vi "01-QNET_MECHKIT_Flexgage.vi"() -> ()   [LabVIEW 2017]
doc: "This VI is to be used with the NI-ELVIS and the QNET-Mechatronic Sensors I module. The objective is to calibrate the strain gage sensor mounted on the flexible link."
uses:
  <vilib>/Simulation/Scripting/Companion Diagram/SimConfigNode/SimParams.ctl
  <vilib>/Simulation/Scripting/Companion Diagram/SimConfigNode/_simSolvers.ctl
  <vilib>/Simulation/Implementation/Shared/SIMSCR Execution Mode.ctl
  <vilib>/Simulation/Param Hierarchy/Typedefs/SIMPH Param Control Actions.ctl
  <vilib>/Simulation/Implementation/Shared/NILVSim_ParamChanged.vi
  <vilib>/Simulation/Implementation/Shared/NILVSIM_BeginStep.vi
  <vilib>/DAQmx/read.llb/DAQmx Read.vi
  <vilib>/DAQmx/read.llb/DAQmx Read (Analog DBL 1Chan 1Samp).vi
  <vilib>/Simulation/Utility/Implementation/NILVSim Collector.llb/SIM Collector (scalar).vi
  <vilib>/Simulation/SignalDisplay/Implementation/NILVSim Time Waveform.llb/SIM Time Waveform (scalar).vi
  <vilib>/Simulation/Utility/Implementation/SIM Halt.vi
  <vilib>/Simulation/Implementation/Shared/NILVSim_Manager.vi
  <vilib>/Utility/error.llb/Clear Errors.vi
  <vilib>/Simulation/Implementation/Shared/NILVSim_FinalizeModel.vi
  <vilib>/Simulation/Utility/Implementation/NILVSim Collector.llb/NILVSim Collector core (scalar).vi
  <vilib>/Simulation/Implementation/Shared/SIM Unbundle Sim Info.vi
  <vilib>/Simulation/Implementation/Shared/NILVSim_Initialize.vi
  <vilib>/Analysis/6fits.llb/Linear Fit.vi
  <vilib>/DAQmx/miscellaneous.llb/DAQmx Fill In Error Info.vi
  <vilib>/Simulation/Utility/Implementation/NILVSim Get Time and IsAcceptedStep.vi
  <vilib>/Simulation/Implementation/Shared/SIMSH Read Queue.vi
  <vilib>/Simulation/Implementation/Shared/NILVSim_GetModelError.vi
  <vilib>/Simulation/Implementation/Shared/SIM Bundle Sim Info.vi
  <vilib>/express/express analysis/Spectral/Block/exnSpectralBlock spectral measurements power poly.vi
  <vilib>/express/express analysis/Spectral/Block/exnSpectralBlock spectral measurements power WFM.vi
  <vilib>/Simulation/Scripting/Companion Diagram/SimConfigNode/SimDog.xnode
  <vilib>/Simulation/Implementation/XNodeFramework/SimXNode/SimX.xnode
  <vilib>/express/express analysis/Spectral/XNode/ExpressSpectralMeasurementsBlockNode.xnode
  <vilib>/Analysis/NI_AALPro.lvlib
  <vilib>/Simulation/Implementation/Shared/NI_SIM_Implementation.lvlib
panel:
  in  "Sampling Rate (Hz)":dbl=100.0 min=0.0 max=1000.0 step=25.0 format="%.1f"
  in  "Device":tag="Dev1"
  in  "Tab Control":T1(tab)
  out "Flexgage (V)":waveform(dbl)(graph)
  in  "Link Position (cm)":dbl[](array[numeric])=[-1.0, -0.5, 0.0, 0.5, 1.0] format="%.1f"
  in  "Sensor Measurement (V)":dbl[](array[numeric])
  out "slope":dbl format="%_3f"
  out "intercept":dbl format="%_3f"
  out "Sensor Readings":T2(graph)
  in  "Offset (cm)":dbl
  in  "Gain (cm/V)":dbl
  out "Flexgage (cm)":waveform(dbl)(graph)
  out "Flexgage (cm) 2":dbl(slide) scale=-1.0..1.0 scale format="%_2f"
  out "Power Spectrum":cluster{"f0":dbl, "df":dbl, "magnitude":dbl[]}(graph)
  in  "stop":bool
  # "QNET-MECHKIT Strain Gage"
  # "NOTE: Place J7 jumper on \"Strain gage\" setting."
  # "1) Move the flexible link at -1.0 cm\n2) Enter measured flexgage sensor values in \"Sensor Measurement (V)\" array.\n3) Repeat for -0.5 cm, 0 cm, 0.5 cm, and 1.0 cm."
  # "Linear curve fitting results:"
  # "Enter gain and offset value for sensor to measure correct position of the flexible link.\n(e.g. display below should read 0.5 cm when ruler is placed at 0.5 cm)."
  # "y = Gain*x + Offset\nwhere\nx is the sensor voltage \ny is the output in centimeters."
  # "1) Perturb the flexible link manually.\n2) Once it stopped resonating, click on the STOP button to stop running the VI.\n3) The spectrum is shown below."
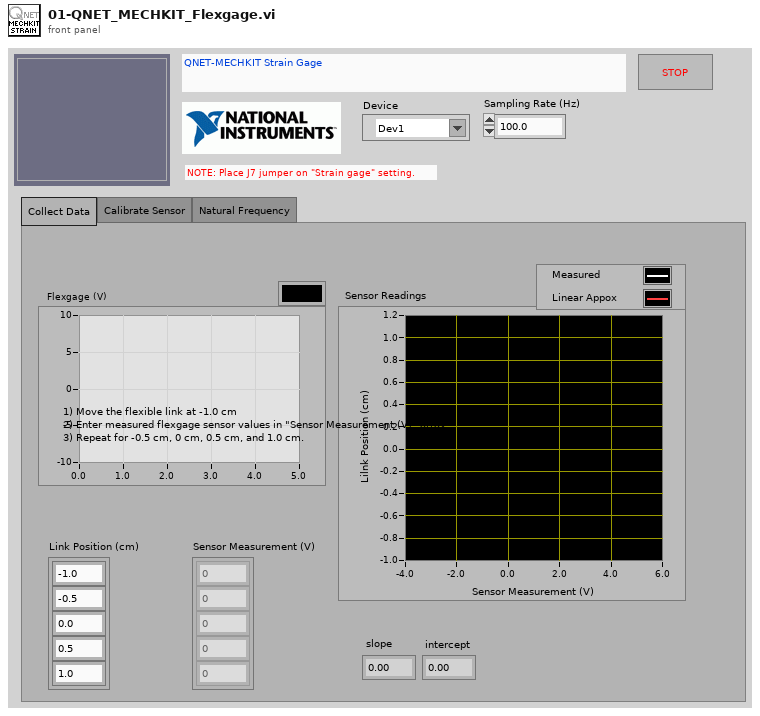
[diagram p1: front panel]
types:
  T1 = enum32{"Collect Data", "Calibrate Sensor", "Natural Frequency"}
  T2 = cluster{"Sensor Measurement (V)":dbl[], "Best Linear Fit":dbl[]}[]
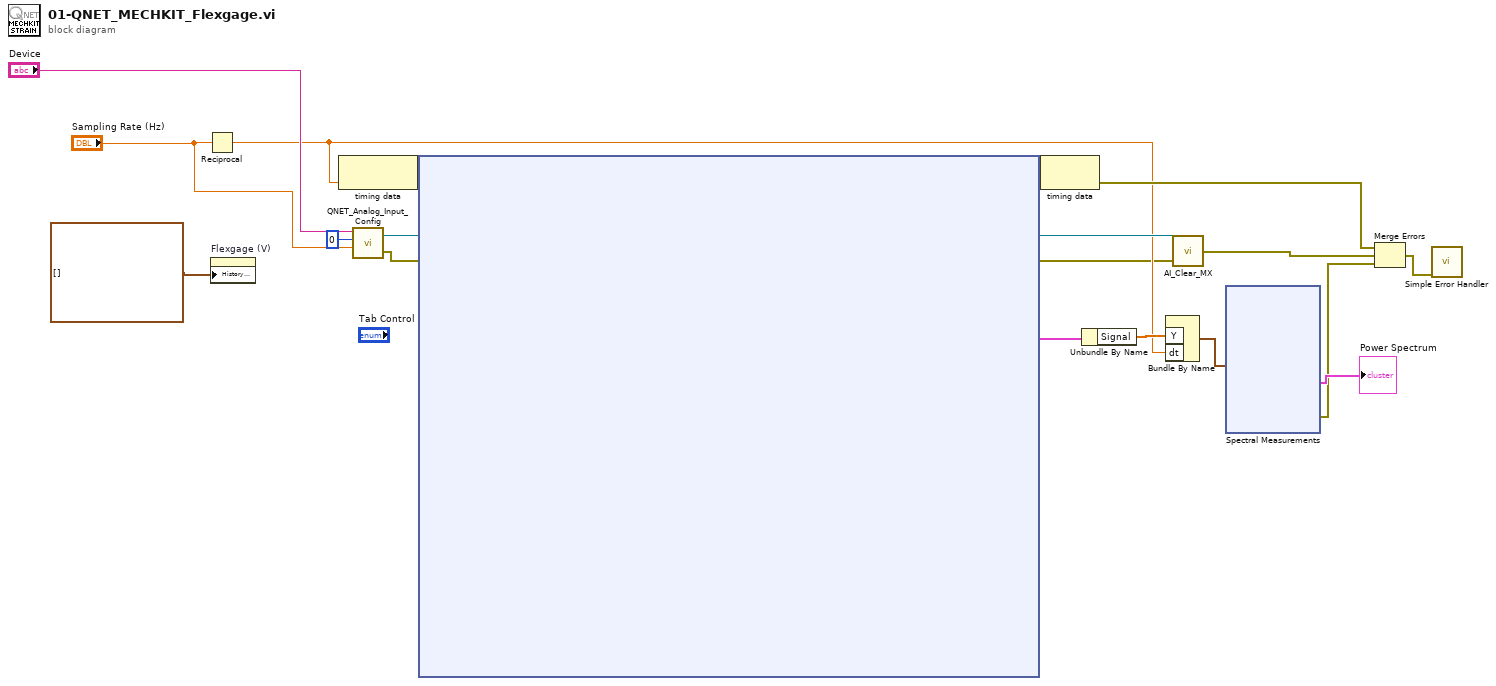
[diagram p0: block diagram]
diagram:
  n1 = Reciprocal(x="Sampling Rate (Hz)") -> (1/x=w5:dbl)
  n2 = property on="Flexgage (V)" class="WFChart (strict)"("History Data"=waveform(dbl)[] []) -> ()  [unwired: 2 in, 2 out]
  n3 = node-c288(w5) -> (w18:variant)
  n4 = call "QNET_Analog_Input_Config.vi"("sampling rate (Hz)"="Sampling Rate (Hz)", "analog input channel"=u32 0, "dev"="Device") -> ("error out"=w15:errorcluster, "task out"=w14:refnum<k21>)  [unwired: 1 in]
  n5 = node-c254 ("Simulation Loop")(w18, w15, w14) -> (w17:variant, w13:refnum<k21>, w2:errorcluster, w7:cluster{"Time":dbl[], "Signal":dbl[]})
  n6 = node-c288(w17) -> (w11:errorcluster)
  n7 = Unbundle By Name(w7) -> ("Signal"=w6:dbl[])
  n8 = Bundle By Name("Y"=w6, "dt"=w5) -> (w4:waveform(dbl))  [unwired: 1 out]
  n9 = call "AI_Clear_MX.vi"("Error in"=w2, "Task in"=w13) -> ("Error out"=w10:errorcluster)
  n10 = xnode "Spectral Measurements"("Signals"=w4) -> ("Power Spectrum"=→"Power Spectrum":cluster{"f0":dbl, "df":dbl, "magnitude":dbl[]}, "error out"=w1:errorcluster)  [unwired: 1 in]
  n11 = Merge Errors(w11, w10, w1) -> (w9:errorcluster)
  n12 = call <vilib>:"Simple Error Handler.vi"("error in (no error)"=w9) -> ()  [unwired: 1 in, 8 out]
